vi "Praks.vi"() -> ()   [LabVIEW 2018]
panel:
  out "Boolean 2":bool
  out "Boolean":bool
  out "Thermometer":dbl(slide) scale=0.0..100.0
  in  "TempMax":dbl(slide) scale=0.0..10.0
  in  "TempMax":dbl(slide) scale=0.0..10.0
  in  "stop":bool
  out "Read String":string
  out "Task":string="GT 0"
  out "Waveform Chart":cluster{"Slide":dbl, "Slide 2":dbl, dbl}(graph)
  in  "VISA resource name":refnum<visa-resource-name>
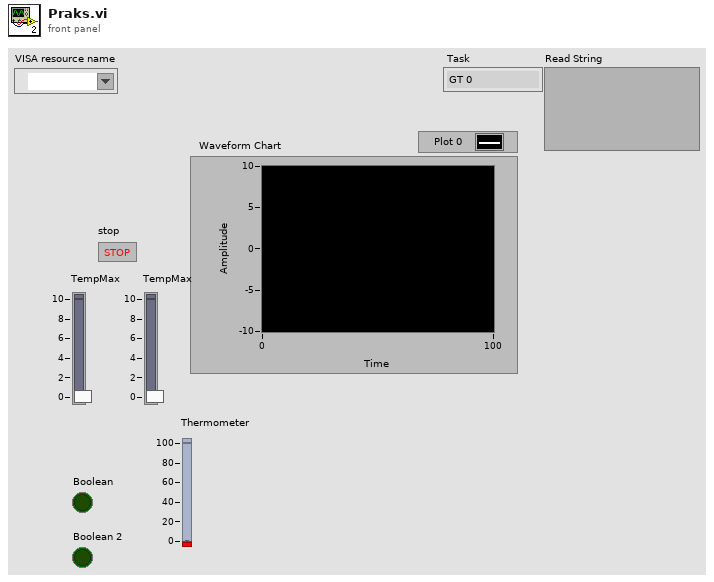
[diagram p1: front panel]
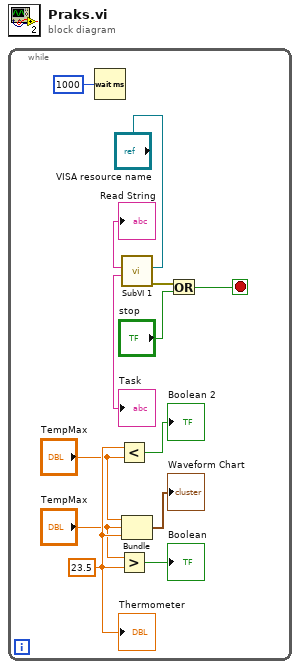
[diagram p0: block diagram]
diagram:
  n1 = while {
    stop <- w7 stop-if-true
    w4 = 23.5
    n2 = Wait (ms)(milliseconds to wait=u32 1000) -> ()  [unwired: 1 out]
    n3 = Less?(x=w4, y="TempMax") -> (x < y?=→"Boolean 2":bool)
    n4 = Greater?(x="TempMax", y=w4) -> (0:→"Boolean":bool)
    n5 = call "SubVI 1.vi"("VISA resource name"="VISA resource name") -> ("error out"=w9:errorcluster, "Task"=→"Task":string, "Read String"=→"Read String":string)  [unwired: 8 in]
    n6 = Bundle("TempMax"="TempMax", "TempMax"="TempMax", w4) -> (→"Waveform Chart":cluster{"TempMax":dbl, "TempMax":dbl, dbl})  [unwired: 1 in]
    n7 = Or(x=w9, y="stop") -> (x .or. y?=w7:bool)
    "Thermometer" <- w4
  }
